vi "glue_dispenser_SingleDot (SubVI).vi"() -> ()   [LabVIEW 2016]
uses:
  <vilib>/LabVIEW Interface for Arduino/Type Defs/Pin Mode.ctl
  <vilib>/Utility/file.llb/Read Delimited Spreadsheet (DBL).vi
  <vilib>/LabVIEW Interface for Arduino/LabVIEW Interface for Arduino.lvlib
panel:
  in  "File to be processed":path=path "C:/Users/Aerotech/Documents/BNL_ThermomechanicalStave/1_ModulePlacement/1_GluePatterning/LabVIEW_gluepattern_array.csv"
  in  "Axis Speeds":T1
  in  "Go to \ncoordinates":T2
  out "DX [s]":dbl format="%#_2g"
  out "DY [s]":dbl format="%#_2g"
  in  "Module width [mm]":dbl
  in  "Module length [mm]":dbl
  out "INPUT":bool[][](array[boolean])
  in  "Duration of glue \ndispensing [s]":dbl
  out "error out":errorcluster
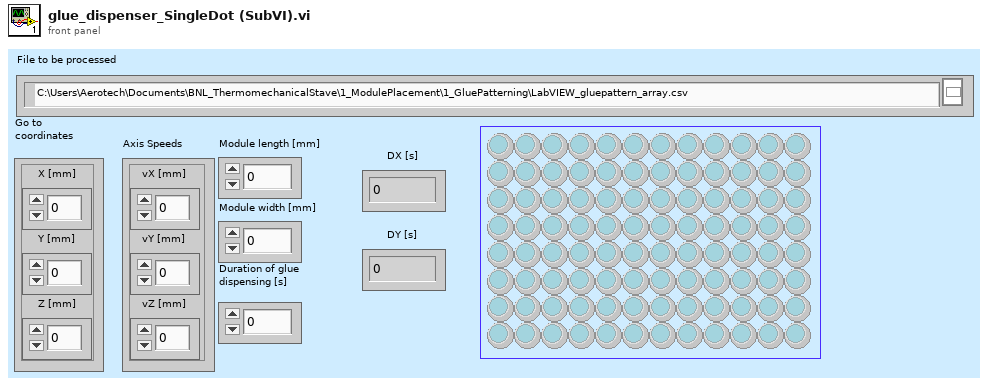
[diagram p1: front panel]
types:
  T1 = cluster{"vX [mm]":dbl, "vY [mm]":dbl, "vZ [mm] ":dbl}
  T2 = cluster{"X [mm]":dbl, "Y [mm]":dbl, "Z [mm] ":dbl}
  T3 = typedef "LabVIEW Interface for Arduino.lvlib/Pin Mode.ctl" = enum8{"Input", "Output"}
  T4 = typedef "LabVIEW Interface for Arduino.lvlib/Arduino Resource.ctl" = cluster{"VISA resource":refnum<visa-resource-name>, "Board Type":T5, "Connection Type":enum8{"USB / Serial"}, "Bytes Per Packet (15)":u8}
  T5 = typedef "LabVIEW Interface for Arduino.lvlib/Board Type.ctl" = enum16{"Uno", "Dimuelanove w/Atmega 328", "Mega 2560"}
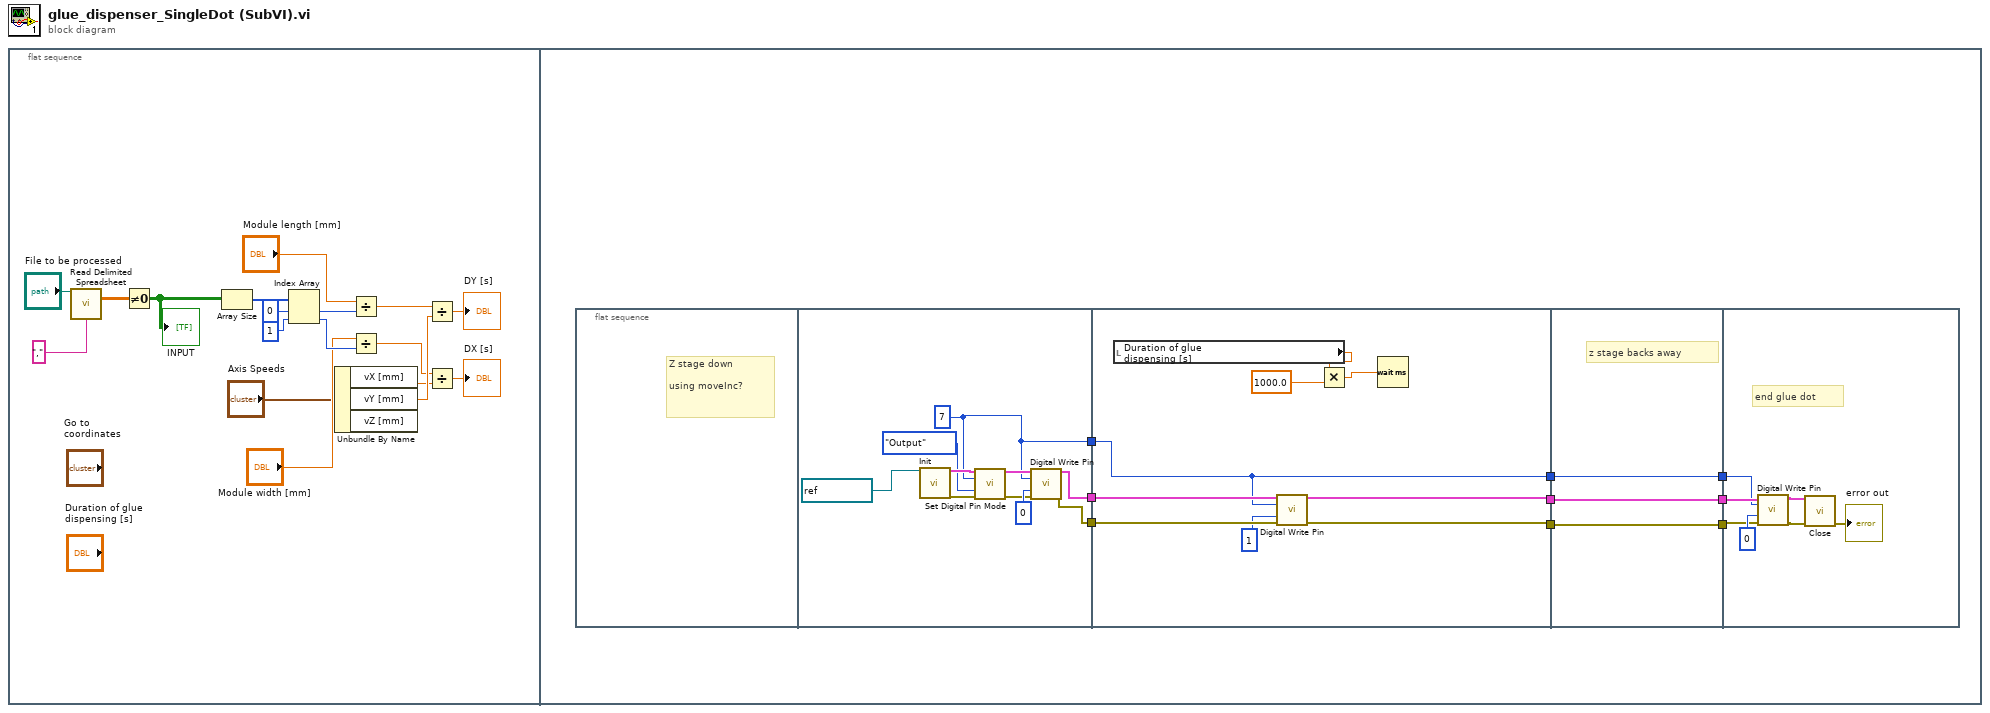
[diagram p0: block diagram]
diagram:
  n1 = flat-sequence {
    frame #0 {
      n2 = call-poly <vilib>:"Read Delimited Spreadsheet.vi"("file path (dialog if empty)"="File to be processed", "delimiter (\\t)"="," ("delimiter (\\t)")) -> ("all rows"=w17:dbl[][])  [unwired: 8 in, 5 out]
      n3 = Not Equal To 0?(x=w17) -> (x != 0?=w16:bool[][])
      "INPUT" <- w16
      n4 = Array Size(array=w16) -> (size(s)=w15:i32[])
      n5 = Index Array(array=w15, index #1=0 ("index"), index #2=1 ("index")) -> (element #1=w11:i32, element #2=w10:i32)
      n6 = Unbundle By Name("Axis Speeds") -> ("vX [mm]"=w5:dbl, "vY [mm]"=w7:dbl)  [unwired: 1 out]
      n7 = Divide(x="Module length [mm]", y=w11) -> (x/y=w8:dbl)
      n8 = Divide(x="Module width [mm]", y=w10) -> (x/y=w4:dbl)
      n9 = Divide(x=w8, y=w7) -> (x/y=→"DY [s]":dbl)
      n10 = Divide(x=w4, y=w5) -> (x/y=→"DX [s]":dbl)
    }
    frame #1 {
      n11 = flat-sequence {
        tunnel: [w29] -> w27
        tunnel: [w28] -> w26
        tunnel: [w30] -> w25
        tunnel: w27 -> [w46]
        tunnel: w26 -> [w45]
        tunnel: w25 -> [w38]
        tunnel: [w44] -> w24
        tunnel: [w43] -> w22
        tunnel: [w38] -> w20
        tunnel: w24 -> [w49]
        tunnel: [w49] -> w23
        tunnel: w22 -> [w48]
        tunnel: [w48] -> w21
        tunnel: w20 -> [w47]
        tunnel: [w47] -> w19
        tunnel: w23 -> [w52]
        tunnel: w21 -> [w50]
        tunnel: w19 -> [w51]
        frame #0 {
          # "Z stage down\n\nusing moveInc?"
        }
        frame #1 {
          w30 = u8 7 ("Digital I/O Pin")
          n12 = call <vilib>:"Init.vi"("VISA resource"=refnum<visa-resource-name> "COM3") -> ("Arduino Resource"=w33:T4, "error out"=w31:errorcluster)  [unwired: 17 in]
          n13 = call <vilib>:"Set Digital Pin Mode.vi"("Arduino Resource"=w33, "Digital I/O Pin"=w30, "Pin Mode (Input)"=Pin_Mode."Output", "error in"=w31) -> ("Arduino Resource"=w35:T4, "error out"=w36:errorcluster)  [unwired: 10 in]
          n14 = call <vilib>:"Digital Write Pin.vi"("Arduino Resource"=w35, "Digital I/O Pin (0)"=w30, "Value (0)"=u8 0, "error in"=w36) -> ("Arduino Resource"=w29:T4, "error out"=w28:errorcluster)  [unwired: 10 in]
        }
        frame #2 {
          n15 = local read "Duration of glue \ndispensing [s]"() -> (w39:dbl)
          n16 = call <vilib>:"Digital Write Pin.vi"("Arduino Resource"=w46, "Digital I/O Pin (0)"=w38, "Value (0)"=u8 1, "error in"=w45) -> ("Arduino Resource"=w44:T4, "error out"=w43:errorcluster)  [unwired: 10 in]
          n17 = Multiply(x=w39, y=1000.0) -> (x*y=w40:dbl)
          n18 = Wait (ms)(milliseconds to wait=w40) -> ()  [unwired: 1 out]
        }
        frame #3 {
          # "z stage backs away"
        }
        frame #4 {
          # "end glue dot"
          n19 = call <vilib>:"Digital Write Pin.vi"("Arduino Resource"=w52, "Digital I/O Pin (0)"=w51, "Value (0)"=u8 0, "error in"=w50) -> ("Arduino Resource"=w54:T4, "error out"=w53:errorcluster)  [unwired: 10 in]
          n20 = call <vilib>:"Close.vi"("Arduino Resource"=w54, "error in"=w53) -> ("error out"=→"error out":errorcluster)  [unwired: 13 in]
        }
      }
    }
  }
